vi "Untitled 22.vi"() -> ()   [LabVIEW 2024]
panel:
  out "error out":errorcluster
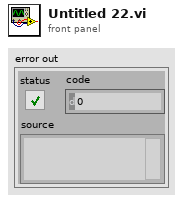
[diagram p1: front panel]
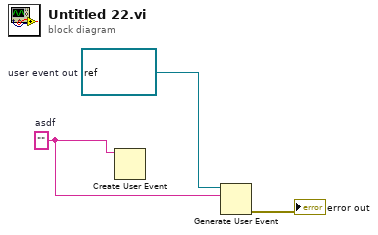
[diagram p0: block diagram]
diagram:
  w3 = refnum<user-event> refnum  # user event out
  w2 = ""  # asdf
  n1 = Create User Event(user event datatype=w2) -> ()  [unwired: 1 in, 2 out]
  n2 = Generate User Event(user event=w3, event data cluster=w2) -> (error out=→"error out":errorcluster)  [unwired: 2 in, 1 out]
